vi "test2dArrayToNx1Array.vi"(8 "error in (no error)":errorcluster) -> (0 "error out":errorcluster)   [LabVIEW 2016]
doc: "Test to transform the 2D NxM array to 1D (N*M)x1 array."
uses:
  <vilib>/addons/_JKI Toolkits/Caraya/classes/Assert/Assert.lvclass
  <vilib>/addons/_JKI Toolkits/Caraya/classes/Test/Test.lvclass
  MatOper/MatOper.lvclass
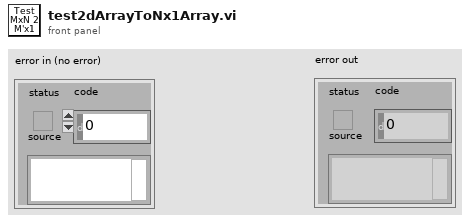
[diagram p1: front panel]
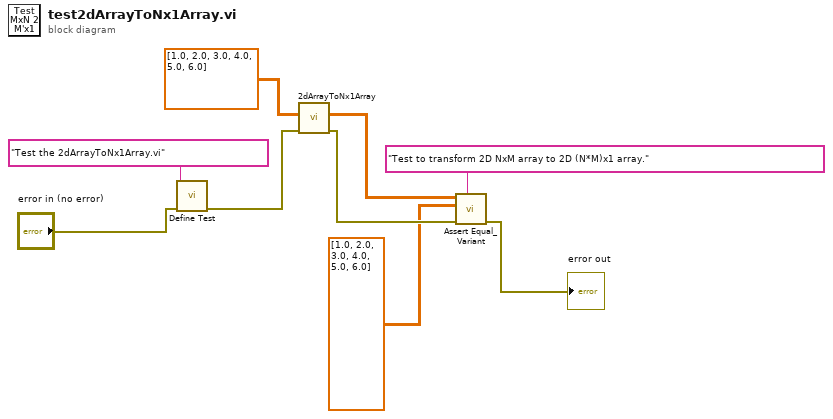
[diagram p0: block diagram]
diagram:
  n1 = call <vilib>:"Define Test.vi"("error in (no error)"="error in (no error)", "Label (VI Title)"="Test the 2dArrayToNx1Array.vi") -> ("error out"=w4:errorcluster)  [unwired: 9 in]
  n2 = call "2dArrayToNx1Array.vi"("error in (no error)"=w4, "2D Array"=dbl[][] [[1.0, 2.0, 3.0], [4.0, 5.0, 6.0]]) -> ("error out"=w2:errorcluster, "nx1 Array"=w3:dbl[][])  [unwired: 7 in, 1 out]
  n3 = call <vilib>:"Assert Equal_Variant.vi"("Label"="Test to transform 2D NxM array to 2D (N*M)x1 array.", "error in (no error)"=w2, "Y"=dbl[][] [[1.0], [2.0], [3.0], [4.0], [5.0], [6.0]], "X"=w3) -> ("error out"=→"error out":errorcluster)  [unwired: 7 in]
